vi "enableTemperatureReading.vi"(8 "error in (no error)":errorcluster, 10 "Enable Temperature (T: Enable)":bool, 11 "Electrometer in":refnum<class "Electrometer.lvclass">) -> (0 "error out":errorcluster, 3 "Electrometer out":refnum<class "Electrometer.lvclass">)   [LabVIEW 2016, in "Electrometer.lvclass"]
uses:
  Electrometer.lvclass
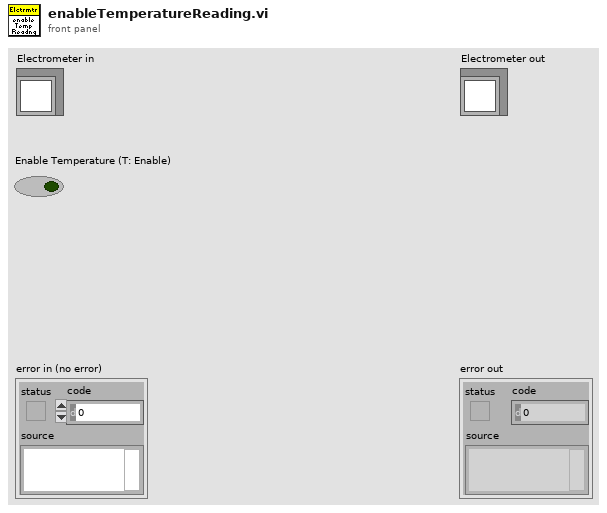
[diagram p1: front panel]
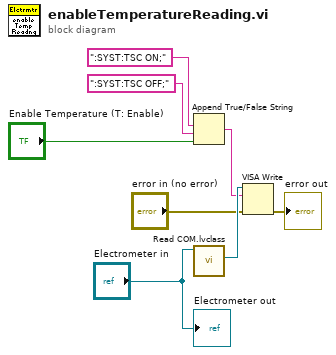
[diagram p0: block diagram]
diagram:
  n1 = Append True/False String(1:"Enable Temperature (T: Enable)", 2:":SYST:TSC OFF;", 3:":SYST:TSC ON;") -> (0:w3:string)  [unwired: 1 in]
  n2 = call "Read COM.lvclass.vi"("Electrometer in"="Electrometer in") -> ("VISA"=w7:refnum<visa-resource-name>)  [unwired: 8 in, 2 out]
  n3 = VISA Write(VISA resource name=w7, write buffer=w3, error in (no error)="error in (no error)") -> (error out=→"error out":errorcluster)  [unwired: 2 out]
  "Electrometer out" <- "Electrometer in"
